vi "test_ThreeSessTwoPinThreeInstrTwoSiteReservation_CallNiDmmGetConnectionsNPinsMConnections_ReturnsThreeConnections.vi"(8 "error in":errorcluster) -> (0 "error out":errorcluster, 2 "result":string, 3 "pass":bool)   [LabVIEW 2020, in "MeasurementServerTests.lvlib"]
uses:
  MeasurementServerTests.lvlib
  Runtime/MeasurementLink Session Management/Session Reservation/Connection.ctl
  Runtime/MeasurementLink Session Management/Session Reservation/Session Reservation.lvclass
  b3e5c3be-b7a7-4b6e-86ee-709eea9cb752.vi
  03fc85e1-696b-4ece-a78b-f41470766ac0.vi
  a536e905-e99b-4ce6-9f7b-add65bd26abc.vi
  f2d0f46c-20cf-4e81-b3a3-5c4fc317eda1.vi
  Runtime/MeasurementLink niDMM/MeasurementLink niDMM.lvlib
  Runtime/MeasurementLink niDMM/Get Connections - NPin MConn.vi
  Runtime/MeasurementLink niDMM/Connection with Session.ctl
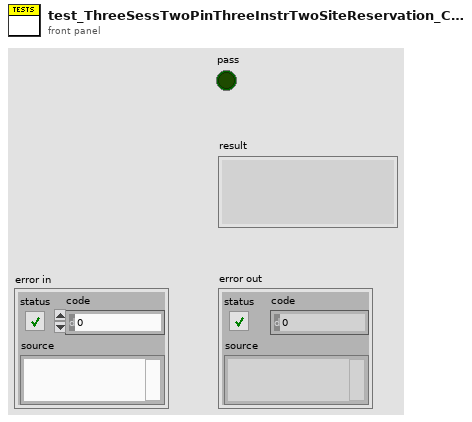
[diagram p1: front panel]
types:
  T1 = typedef "MeasurementLink niDMM.lvlib/Connection with Session.ctl" = cluster{"connection":T2, "session":refnum<k15>}
  T2 = typedef "MeasurementLink Session Management.lvlib/Session Reservation.lvclass/Connection.ctl" = cluster{"pin or relay name":string, "site":i32, "instrument type id":string, "channel":string}
  T3 = typedef "MeasurementLink Session Management.lvlib/Session Reservation.lvclass/Data.ctl" = cluster{"session and driver infos":T4[], "pin or relay names":string[], "connection map":refnum<class "Connection Map.lvclass">, "pin map context":T8, "reservation observer":refnum<class "IReservationObserver.lvclass">, "dvr valid":bool}
  T4 = typedef "MeasurementLink Session Management.lvlib/Session Reservation.lvclass/Session and Driver Info.ctl" = cluster{"session info":T5, "session":variant, "instrument":refnum<class "IInstrument.lvclass">}
  T5 = typedef "MeasurementLink Session Management Client.lvlib/ni_measurementlink_sessionmanagement_v1_SessionInformation.ctl" = cluster{"session":T6, "resource_name":string, "channel_list":string, "instrument_type_id":string, "session_exists":bool, "channel_mappings":T7[]}
  T6 = typedef "MeasurementLink Session Management Client.lvlib/nidevice_grpc_Session.ctl" = cluster{"name":string}
  T7 = typedef "MeasurementLink Session Management Client.lvlib/ni_measurementlink_sessionmanagement_v1_ChannelMapping.ctl" = cluster{"pin_or_relay_name":string, "site":i32, "channel":string}
  T8 = typedef "MeasurementLink Session Management Client.lvlib/ni_measurementlink_PinMapContext.ctl" = cluster{"pin_map_id":string, "sites":i32[]}
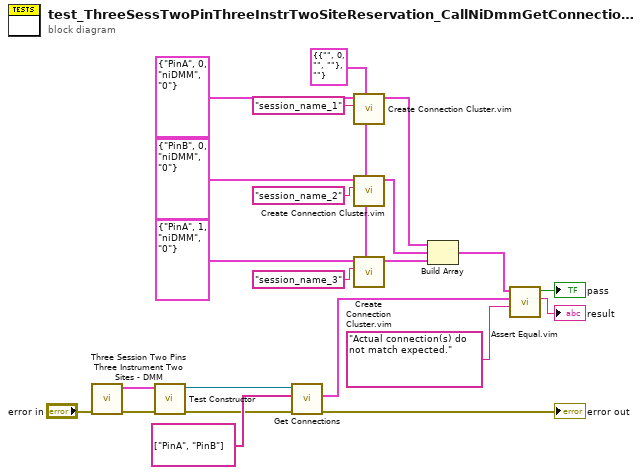
[diagram p0: block diagram]
diagram:
  w5 = T1 {"connection"={"pin or relay name"="", "site"=0, "instrument type id"="", "channel"=""}, "session"=""} ("connection with session")
  n1 = call "Three Session Two Pins Three Instrument Two Sites - DMM.vi"("error in"="error in") -> ("error out"=w7:errorcluster, "data out"=w8:T3)  [unwired: 9 in]
  n2 = call "Test Constructor.vi"("error in"=w7, "data"=w8) -> ("error out"=w11:errorcluster, "Session Reservation out"=w13:refnum<class "Session Reservation.lvclass">)  [unwired: 8 in]
  n3 = call-poly "Get Connections.vi"("error in"=w11, "pin or relay names"=string[] ["PinA", "PinB"], "session reservation in"=w13) -> ("error out"=→"error out":errorcluster, "connections"=w9:T1[])  [unwired: 6 in, 1 out]
  n4 = call "Create Connection Cluster.vim"("connection type"=w5, "session in"="session_name_1", "hardware independent connection in"=T2 {"pin or relay name"="PinA", "site"=0, "instrument type id"="niDMM", "channel"="0"} ("connection")) -> ("connection out"=w18:T1)  [unwired: 8 in]
  n5 = call "Create Connection Cluster.vim"("connection type"=w5, "session in"="session_name_2", "hardware independent connection in"=T2 {"pin or relay name"="PinB", "site"=0, "instrument type id"="niDMM", "channel"="0"} ("connection")) -> ("connection out"=w17:T1)  [unwired: 8 in]
  n6 = call "Create Connection Cluster.vim"("connection type"=w5, "session in"="session_name_3", "hardware independent connection in"=T2 {"pin or relay name"="PinA", "site"=1, "instrument type id"="niDMM", "channel"="0"} ("connection")) -> ("connection out"=w14:T1)  [unwired: 8 in]
  n7 = Build Array(w18, w17, w14) -> (w16:T1[])
  n8 = call "Assert Equal.vim"("failure message"="Actual connection(s) do not match expected.", "actual value"=w9, "expected value"=w16) -> ("message"=→"result":string, "equal?"=→"pass":bool)  [unwired: 7 in]
